vi "_TangoReadAttributes.vi"(2 "error in":errorcluster, 3 "attribute names":string[](array[string]), 4 "device name":string) -> (0 "error out":errorcluster, 1 "attribute values":T1[](array[typedef]))   [LabVIEW 2014, in "tango.lvlib"]
uses:
  tango.lvlib
  Common VIs/Typedefs/_AttributeQuality_t.ctl
  Common VIs/Typedefs/_AttributeDataType_t.ctl
  Common VIs/Typedefs/_AttributeValue_t.ctl
  tango_binding.dll
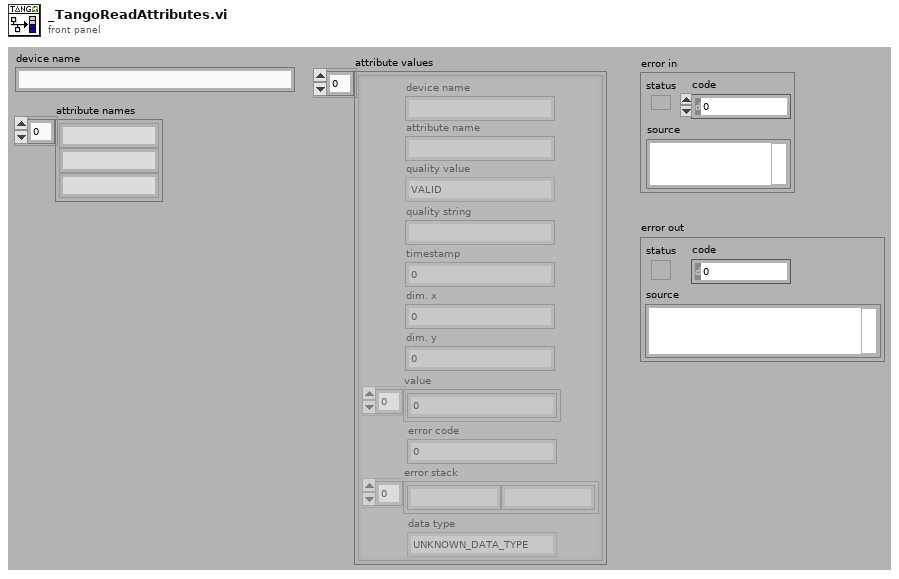
[diagram p1: front panel]
types:
  T1 = typedef "tango.lvlib/_AttributeValue_t.ctl" = cluster{"device name":string, "attribute name":string, "quality value":T2, "quality string":string, "timestamp":dbl, "dim. x":i32, "dim. y":i32, "value":u8[], "error code":i32, "error stack":string[], "data type":T3}
  T2 = typedef "tango.lvlib/_AttributeQuality_t.ctl" = enum16{"VALID", "INVALID", "ALARM", "CHANGING", "UNKNOWN_QUALITY"}
  T3 = typedef "tango.lvlib/_AttributeDataType_t.ctl" = enum16{"STATE_SCA", "STATE_SPE", "STATE_IMG", "STRING_SCA", "STRING_SPE", "STRING_IMG", "BOOL_SCA", "BOOL_SPE", "BOOL_IMG", "UCHAR_SCA", "UCHAR_SPE", "UCHAR_IMG", "SHORT_SCA", "SHORT_SPE", "SHORT_IMG", "USHORT_SCA", "USHORT_SPE", "USHORT_IMG", "LONG_SCA", "LONG_SPE", "LONG_IMG", "ULONG_SCA", "ULONG_SPE", "ULONG_IMG", "LONG64_SCA", "LONG64_SPE", "LONG64_IMG", "ULONG64_SCA", "ULONG64_SPE", "ULONG64_IMG", "FLOAT_SCA", "FLOAT_SPE", "FLOAT_IMG", "DOUBLE_SCA", "DOUBLE_SPE", "DOUBLE_IMG", "ENUM_SCA", "UNKNOWN_DATA_TYPE"}
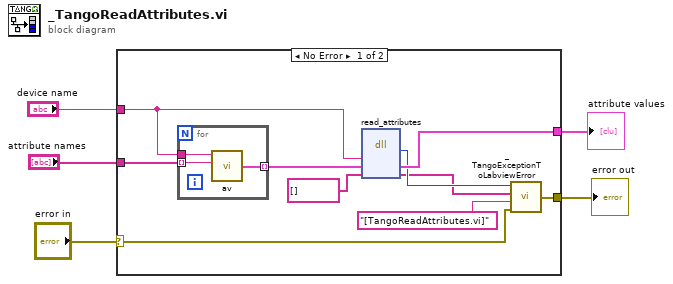
[diagram p0: block diagram]
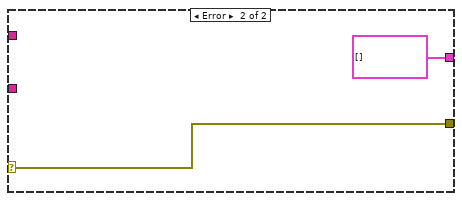
[diagram p2: hidden frame]
diagram:
  n1 = case shown="No Error" "error in" {
    selector: "error in" -> [w6 w20]
    tunnel: "attribute names" -> [w15 _]
    tunnel: "device name" -> [w14 _]
    tunnel: [w11 T1[] [] ("attr_values_inout")] -> w3
    tunnel: [w7 w20] -> w1
    frame No Error {
      n2 = for {
        tunnel: w14 -> [w17]
        tunnel: w15 -> [w16] mode=indexing
        tunnel: [w18] -> w12 mode=indexing
        n3 = call "av.vi"("attribute name"=w16, "device name"=w17) -> ("attribute value"=w18:T1)  [unwired: 4 in]
      }
      n4 = dll-call lib="tango_binding.*" fn="read_attributes"("dev_name"=w14, "attr_values_inout"=w12, "error_stack"=string[] [] ("error stack")) -> ("return type"=w9:i32, "attr_values_inout"=w11:T1[], "error_stack"=w8:string[])  [unwired: 4 in, 2 out]
      n5 = call "_TangoExceptionToLabviewError.vi"("error in"=w6, "location"="[TangoReadAttributes.vi]", "error stack"=w8, "error code"=w9) -> ("error out"=w7:errorcluster)
    }
    frame Error {
    }
  }
  "attribute values" <- w3
  "error out" <- w1
